vi "Handle Error.vi"(8 "error in (no error)":errorcluster, 11 "Elevator Controller in":refnum<class "Elevator Controller.lvclass">) -> (0 "error out":errorcluster, 2 "stop actor?":bool=TRUE, 3 "Elevator Controller out":refnum<class "Elevator Controller.lvclass">)   [LabVIEW 2022 SP3, in "Elevator Controller.lvlib" / "Elevator Controller.lvclass"]
doc: "(<B>Filename</B>: Actor Framework.lvlib:Actor.lvclass:Handle Error.vi)\n\nDefines how the actor handles an error that occurred while processing a message.\n\nBy default, this method does nothing except stop the actor. This method also treats error code 43 (coming from <B>error in</B>) as a sign that the actor shut down normally. In this situation, the Handle Error method does not return the error on <B>error out</B>, meaning the actor's caller will not receive it. All other error codes will be returned on <B>error out</B>.\n\nA descendant class may override this method to change this behavior."
uses:
  Elevator Controller.lvclass
  C:/Program Files/National Instruments/LabVIEW 2022/vi.lib/ActorFramework/Actor/Actor.lvclass
  States -Enum.ctl
  <vilib>/ActorFramework/Actor/Actor.lvclass/Actor.ctl
  <vilib>/ActorFramework/Message Enqueuer/Message Enqueuer.lvclass/Message Enqueuer.ctl
  Elevator Controller Messages/Centralize Error Msg/Centralize Error Msg.lvclass/Centralize Error Msg.ctl
  Elevator Controller Messages/Set State Msg/Set State Msg.lvclass/Set State Msg.ctl
  <vilib>/ActorFramework/Message Enqueuer/Init from Existing Queue.vi
  <vilib>/ActorFramework/Message Enqueuer/Enqueue.vi
  Elevator Controller Messages/Centralize Error Msg/Centralize Error Msg.lvclass
  C:/Program Files/National Instruments/LabVIEW 2022/vi.lib/ActorFramework/Message/Message.lvclass
  Elevator Controller Messages/Set State Msg/Set State Msg.lvclass
  <vilib>/ActorFramework/Message Priority Queue/Priority Enqueue.vi
  <vilib>/ActorFramework/Actor/Actor.lvclass
  <vilib>/ActorFramework/Message Enqueuer/Message Enqueuer.lvclass
  Elevator Controller.lvclass/Elevator Controller.ctl
  Incoming Messages/Set State Msg/Set State Msg.lvclass
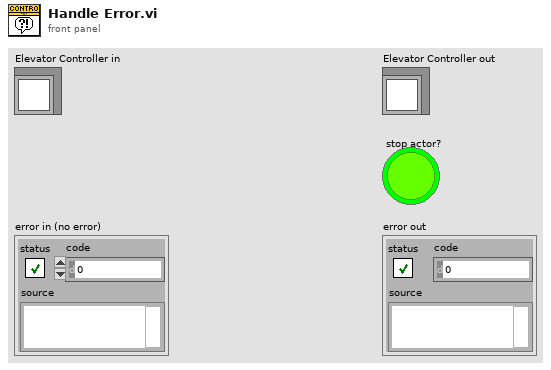
[diagram p1: front panel]
types:
  T1 = typedef "Elevator Controller.lvlib/Elevator Controller.lvclass/States -Enum.ctl" = enum16{"Initial State", "Wait for First Request", "Start and Move State", "Analysis State", "Continue Travel State", "Stop at Floor", "Open and Close Door Sequence", "No Request Remaining", "Emergency Call", "Terminate Process", ""}
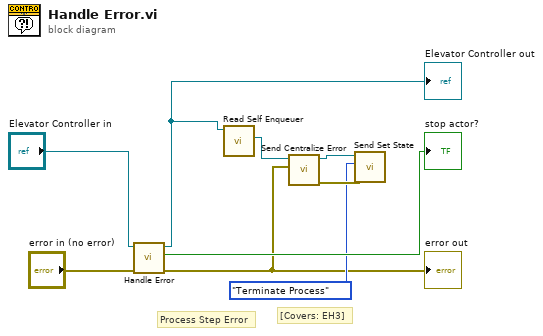
[diagram p0: block diagram]
diagram:
  # "Process Step Error"
  # "[Covers: EH3]"
  n1 = call-parent "Handle Error.vi"("error in (no error)"="error in (no error)", "Actor in"="Elevator Controller in") -> ("error out"=w1:errorcluster, "stop actor?"=→"stop actor?":bool, "Actor out"=w3:refnum<class "Elevator Controller.lvclass">)  [unwired: 7 in]
  "Elevator Controller out" <- w3
  "error out" <- w1
  n2 = call <vilib>:"Read Self Enqueuer.vi"("Actor"=w3) -> ("Self Enqueuer"=w2:refnum<class "Message Enqueuer.lvclass">)  [unwired: 10 in]
  n3 = call "Send Centralize Error.vi"("Error"=w1, "Message Enqueuer"=w2) -> ("error out"=w5:errorcluster, "Message Enqueuer out"=w6:refnum<class "Message Enqueuer.lvclass">)  [unwired: 8 in]
  n4 = call "Send Set State.vi"("error in (no error)"=w5, "State"=States_-Enum."Terminate Process" ("Enum"), "Message Enqueuer"=w6) -> ()  [unwired: 7 in, 2 out]
